vi "Accumulate.vi"(0 "Input":i32, 1 "Reset? (F)":bool) -> (2 "Accumulation":i32)   [LabVIEW 2014]
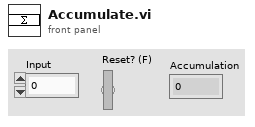
[diagram p1: front panel]
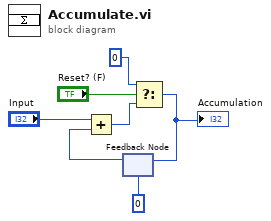
[diagram p0: block diagram]
diagram:
  n1 = feedback #1(0 ("t")) -> (w2:i32)
  n2 = Add(x="Input", y=w2) -> (x+y=w6:i32)
  n3 = Select(t=0, s="Reset? (F)", f=w6) -> (s? t:f=w3:i32)
  "Accumulation" <- w3
  n4 = feedback-in #1(w3) -> ()
